vi "_emi_Find VIs in mem with version info.vi"(11 "error in (no error)":errorcluster) -> (8 "VIs with Version VIs on top lvl diagram":string[](array[string]), 15 "error out":errorcluster)   [LabVIEW 2010]
doc: "Get a list of the Vis in memory where emi: \"_Set Application version from Containing VI.vi\" i\\s on top level diagram."
uses:
  <vilib>/UserTags/UserTags.lvlib
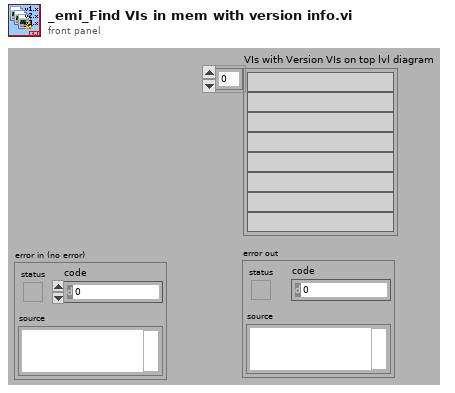
[diagram p1: front panel]
types:
  T1 = enum32{"invalid VI type", "Standard VI", "Control VI", "Global VI", "Polymorphic VI", "Configuration VI", "SubSystem", "Facade VI", "Method VI", "Statechart Diagram VI"}
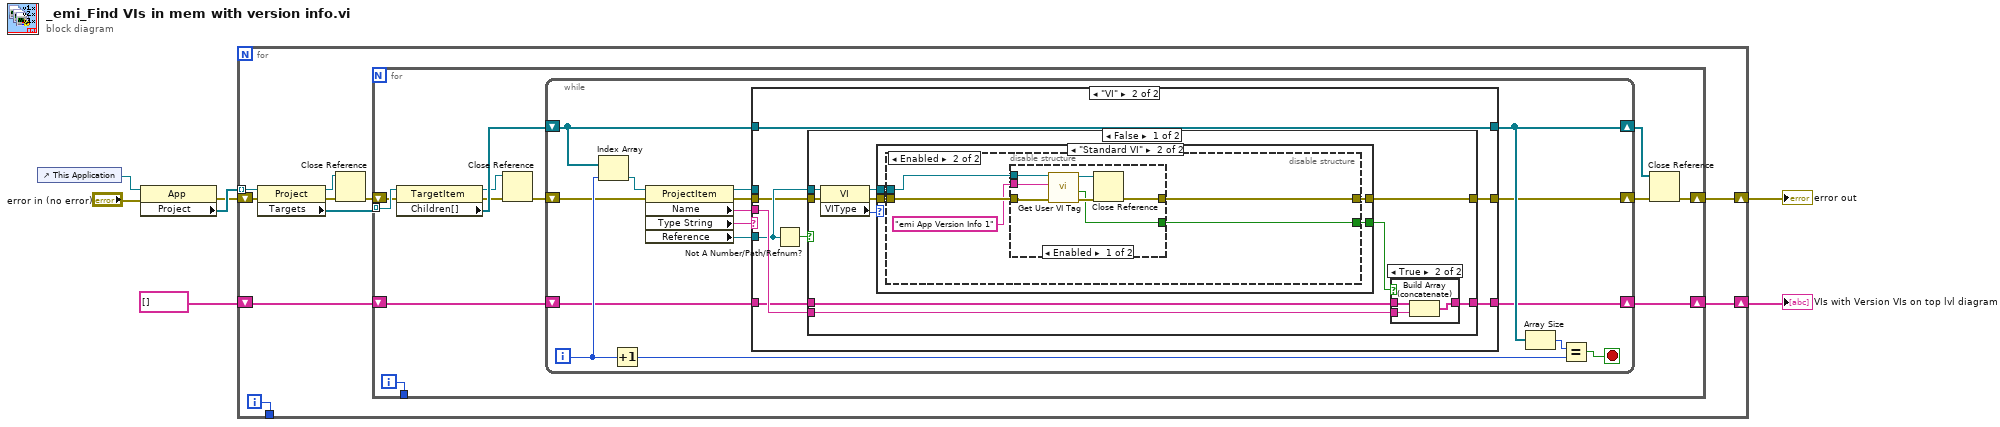
[diagram p0: block diagram]
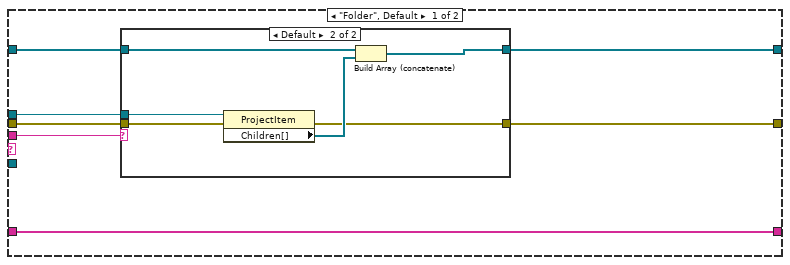
[diagram p2: hidden frame]
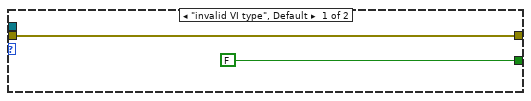
[diagram p4: hidden frame]
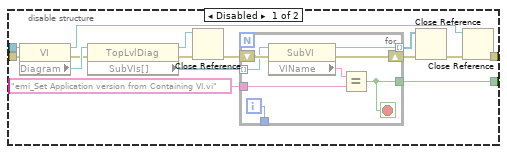
[diagram p5: hidden frame]
diagram:
  n1 = control-ref of="This Application"() -> (w4:refnum<vi>)
  n2 = property class="App"(reference=w4, error in="error in (no error)") -> (error out=w2:errorcluster, "Project"=w7:refnum<vi>[])  [unwired: 1 out]
  n3 = for {
    tunnel: w7 -> [w17] mode=indexing
    shift-right: [w14] -> w5
    shift-left: string[] [] ("Application:All VIs In Memory") -> [w15]
    shift-right: [w9] -> w1
    shift-left: w2 -> [w13]
    tunnel: [w8] -> _
    i -> [w8]
    n4 = property class="Project"(reference=w17, error in=w13) -> (reference out=w11:refnum<vi>, error out=w12:errorcluster, "Targets"=w16:refnum<vi>[])
    n5 = Close Reference(reference=w11, error in (no error)=w12) -> (error out=w10:errorcluster)
    n6 = for {
      tunnel: w16 -> [w29] mode=indexing
      shift-right: [w26] -> w14
      shift-left: w15 -> [w27]
      shift-right: [w19] -> w9
      shift-left: w10 -> [w25]
      tunnel: [w18] -> _
      i -> [w18]
      n7 = property class="TargetItem"(reference=w29, error in=w25) -> (reference out=w23:refnum<vi>, error out=w24:errorcluster, "Children[]"=w28:refnum<vi>[])
      n8 = Close Reference(reference=w23, error in (no error)=w24) -> (error out=w22:errorcluster)
      n9 = while {
        shift-right: [w40] -> w20
        shift-left: w28 -> [w42]
        shift-right: [w33] -> w26
        shift-left: w27 -> [w34]
        shift-right: [w30] -> w21
        shift-left: w22 -> [w32]
        i -> [w38]
        stop <- w37 stop-if-true
        n10 = Index Array(array=w42, index=w38) -> (element=w43:refnum<vi>)
        n11 = Increment(x=w38) -> (x+1=w36:i32)
        n12 = property class="ProjectItem"(reference=w43, error in=w32) -> (reference out=w41:refnum<vi>, error out=w31:errorcluster, "Name"=w45:string, "Type String"=w44:string, "Reference"=w35:refnum<vi>)
        n13 = case shown="\"VI\"" w44 {
          tunnel: w45 -> [w49 w68]
          tunnel: [w51 w67] -> w40
          tunnel: w42 -> [w52 w67]
          tunnel: w41 -> [w50 _]
          tunnel: w35 -> [_ w66]
          tunnel: w34 -> [w48 w64]
          tunnel: [w48 w63] -> w33
          tunnel: w31 -> [w47 w62]
          tunnel: [w46 w61] -> w30
          frame "Folder", Default {
            n14 = case shown="Default" w49 {
              tunnel: w52 -> [w54 w60]
              tunnel: [w54 w59] -> w51
              tunnel: w50 -> [_ w58]
              tunnel: w47 -> [w53 w56]
              tunnel: [w53 w55] -> w46
              frame "Dependencies" {
              }
              frame Default {
                n15 = property class="ProjectItem"(reference=w58, error in=w56) -> (error out=w55:errorcluster, "Children[]"=w57:refnum<vi>[])  [unwired: 1 out]
                n16 = Build Array (concatenate)(w60, w57) -> (w59:refnum<vi>[])
              }
            }
          }
          frame "VI" {
            n17 = Not A Number/Path/Refnum?(number/path/refnum=w66) -> (NaN/Path/Refnum?=w65:bool)
            n18 = case shown="False" w65 {
              tunnel: w68 -> [w73 _]
              tunnel: w66 -> [w77 _]
              tunnel: w64 -> [w76 w126]
              tunnel: [w75 w126] -> w63
              tunnel: w62 -> [w72 w125]
              tunnel: [w71 w125] -> w61
              frame False {
                n19 = property class="VI"(reference=w77, error in=w72) -> (reference out=w69:refnum<vi>, error out=w78:errorcluster, "VIType"=w70:T1)
                n20 = case shown="\"Standard VI\"" w70 {
                  tunnel: w78 -> [w80 w83]
                  tunnel: [FALSE w84] -> w74
                  tunnel: [w80 w81] -> w71
                  tunnel: w69 -> [_ w82]
                  frame "invalid VI type", Default {
                  }
                  frame "Standard VI" {
                    n21 = disable-structure shown="Enabled" {
                      disable-tunnel: [w97 w110] -> w84
                      disable-tunnel: w83 -> [w96 w111]
                      disable-tunnel: w82 -> [w95 w109]
                      disable-tunnel: [w87 w112] -> w81
                      frame Disabled {
                        n22 = property class="VI"(reference=w95, error in=w96) -> (reference out=w85:refnum<vi>, error out=w88:errorcluster, "Diagram"=w94:refnum<vi>)
                        n23 = property class="TopLvlDiag"(reference=w94, error in=w88) -> (reference out=w92:refnum<vi>, error out=w93:errorcluster, "SubVIs[]"=w99:refnum<vi>[])
                        n24 = Close Reference(reference=w92, error in (no error)=w93) -> (error out=w91:errorcluster)
                        n25 = for {
                          tunnel: w99 -> [w105] mode=indexing
                          tunnel: "emi_Set Application version from Containing VI.vi" -> [w103]
                          tunnel: [w102] -> w97
                          tunnel: [w101] -> _
                          shift-right: [w106] -> w90
                          shift-left: w91 -> [w107]
                          tunnel: [w100] -> w89 mode=indexing
                          i -> [w101]
                          stop <- w102 stop-if-true
                          n26 = property class="SubVI"(reference=w105, error in=w107) -> (reference out=w100:refnum<vi>, error out=w106:errorcluster, "VIName"=w104:string)
                          n27 = Equal?(x=w104, y=w103) -> (x = y?=w102:bool)
                        }
                        n28 = Close Reference(reference=w89, error in (no error)=w90) -> (error out=w86:errorcluster)
                        n29 = Close Reference(reference=w85, error in (no error)=w86) -> (error out=w87:errorcluster)
                      }
                      frame Enabled {
                        n30 = disable-structure shown="Enabled" {
                          disable-tunnel: [w119 w120] -> w112
                          disable-tunnel: w111 -> [w118 w120]
                          disable-tunnel: [w116 _] -> w110
                          disable-tunnel: w109 -> [w114 _]
                          disable-tunnel: "emi App Version Info 1" ("Tag Name") -> [w113 _]
                          frame Enabled {
                            n31 = call <vilib>:"Get User VI Tag.vi"("error in (no error)"=w118, "Tag Name"=w113, "VI Refnum"=w114) -> ("error out"=w117:errorcluster, "Was Tag Found?"=w116:bool, "dup VI Refnum"=w115:refnum<vi>)  [unwired: 5 in, 1 out]
                            n32 = Close Reference(reference=w115, error in (no error)=w117) -> (error out=w119:errorcluster)
                          }
                          frame Disabled {
                          }
                        }
                      }
                    }
                  }
                }
                n33 = case shown="True" w74 {
                  tunnel: w76 -> [w121 w124]
                  tunnel: [w121 w123] -> w75
                  tunnel: w73 -> [_ w122]
                  frame False {
                  }
                  frame True {
                    n34 = Build Array (concatenate)(w124, w122) -> (w123:string[])
                  }
                }
              }
              frame True {
              }
            }
          }
        }
        n35 = Array Size(array=w40) -> (size(s)=w39:i32)
        n36 = Equal?(x=w39, y=w36) -> (x = y?=w37:bool)
      }
      n37 = Close Reference(reference=w20, error in (no error)=w21) -> (error out=w19:errorcluster)
    }
  }
  "VIs with Version VIs on top lvl diagram" <- w5
  "error out" <- w1
